vi "Autonomous Independent.vi"   [LabVIEW 2018]
doc: "This VI is called when autonomous begins, and will automatically be terminated when autonomous ends. You can carry out timed or sensor driven robot movement independently without needing to return to the caller."
uses:
  <vilib>/Rock Robotics/Network Tables/NT Read String.vi
  RobotGlobal.vi
  Classes/Pnematics control/Pneumatics.lvclass
  Classes/Pnematics control/Solenoids/Solenoids.lvclass
panel:
  # "Be sure to right-click and choose Data Operations>>Make Current Value default if you want to save the array values with the VI"
types:
  T1 = typedef "RobotObjects.ctl" = cluster{"Drive.lvclass":refnum<class "Drive.lvclass">, "Pneumatics.lvclass":refnum<class "Pneumatics.lvclass">, "Vision.lvclass":refnum<class "Vision.lvclass">, "Joysticks.lvclass":refnum<class "Joysticks.lvclass">, "Elevator.lvclass":refnum<class "Elevator.lvclass">, "Hatch.lvclass":refnum<class "Hatch.lvclass">, "Cargo.lvclass":refnum<class "Cargo.lvclass">}
  T2 = typedef "Pneumatics control.lvlib/Pneumatics.lvclass/Solenoids.ctl" = cluster{"DriveShift":refnum<class "Solenoids.lvclass">, "Vacuum":refnum<class "Solenoids.lvclass">, "HatchArm":refnum<class "Solenoids.lvclass">, "HatchGrabber":refnum<class "Solenoids.lvclass">}
  T3 = cluster{"[0]":refnum<class "Solenoids.lvclass">, "[1]":refnum<class "Solenoids.lvclass">, "[2]":refnum<class "Solenoids.lvclass">, "[3]":refnum<class "Solenoids.lvclass">}
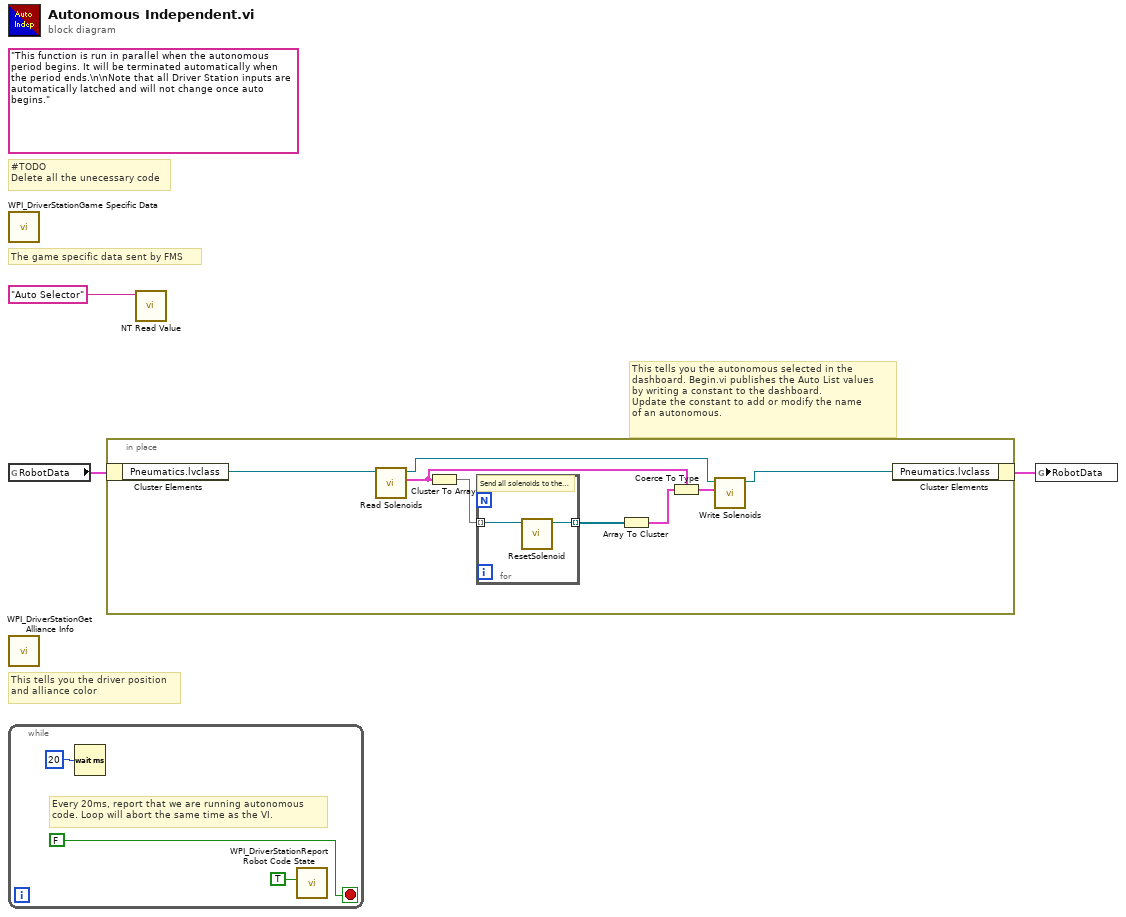
[diagram p0: block diagram]
diagram:
  (unwired) "This function is run in parallel when the autonomous period begins. It will be terminated automatically when the period ends.\n\nNote that all Driver Station inputs are automatically latched and will not change once auto begins."
  # "#TODO\nDelete all the unecessary code"
  # "The game specific data sent by FMS"
  # "This tells you the autonomous selected in the \ndashboard. Begin.vi publishes the Auto List values\nby writing a constant to the dashboard.\nUpdate the constant to add or modify the name\nof an autonomous."
  # "This tells you the driver position\nand alliance color"
  n1 = call <vilib>:"WPI_DriverStationGame Specific Data.vi"() -> ()  [unwired: 11 in, 1 out]
  n2 = global read "RobotGlobal.vi" "RobotData"() -> (w2:T1)
  n3 = call <vilib>:"WPI_DriverStationGet Alliance Info.vi"() -> ()  [unwired: 12 out]
  n4 = while {
    stop <- FALSE stop-if-true
    # "Every 20ms, report that we are running autonomous\ncode. Loop will abort the same time as the VI."
    n5 = Wait (ms)(milliseconds to wait=u32 20) -> ()  [unwired: 1 out]
    n6 = call <vilib>:"WPI_DriverStationReport Robot Code State.vi"("Autonomous"=TRUE) -> ()  [unwired: 10 in, 1 out]
  }
  n7 = in-place {
    n8 = in-place-cluster #1(w2) -> ("Pneumatics.lvclass"=w8:refnum<class "Pneumatics.lvclass">)
    n9 = call-dynamic "Read Solenoids.vi"("Pneumatics in"=w8) -> ("Solenoids"=w9:T2, "Pneumatics out"=w14:refnum<class "Pneumatics.lvclass">)  [unwired: 8 in, 1 out]
    n10 = Cluster To Array(cluster=w9) -> (array=w13:refnum<class "Solenoids.lvclass">[])
    n11 = for {
      tunnel: [w16] -> w12 mode=indexing
      tunnel: w13 -> [w15] mode=indexing
      # "Send all solenoids to the correct position"
      n12 = call-dynamic "ResetSolenoid.vi"("Solenoids in"=w15) -> ("Solenoids out"=w16:refnum<class "Solenoids.lvclass">)  [unwired: 9 in, 1 out]
    }
    n13 = Array To Cluster(array=w12) -> (cluster=w11:T3)
    n14 = Coerce To Type(0:w11, 1:w9) -> (2:w10:T2)
    n15 = call-dynamic "Write Solenoids.vi"("Solenoids"=w10, "Pneumatics in"=w14) -> ("Pneumatics out"=w7:refnum<class "Pneumatics.lvclass">)  [unwired: 8 in, 1 out]
    n16 = in-place-cluster #1("Pneumatics.lvclass"=w7) -> (w1:T1)
  }
  n17 = call-poly <vilib>:"NT Read Value.vi"("Name"="Auto Selector") -> ()  [unwired: 9 in, 2 out]
  n18 = global write "RobotGlobal.vi" "RobotData"(w1) -> ()
